vi "FTW-Test-JSON-FloatingPoint.vi"() -> (0 "Test Result":errorcluster)   [LabVIEW 2015]
uses:
  src/json/FTW-JSON-Type.ctl
  src/error/FTW-ERR-ThrowInfo.vi
  src/error/FTW-ERR-ThrowError.vi
  src/error/FTW-ERR-CallChain.vi
  src/string/FTW-STR-ReplaceWhitespace.vi
  src/string/FTW-STR-Array-Delimit.vi
panel:
  out "JSON String (UTF-8)":string
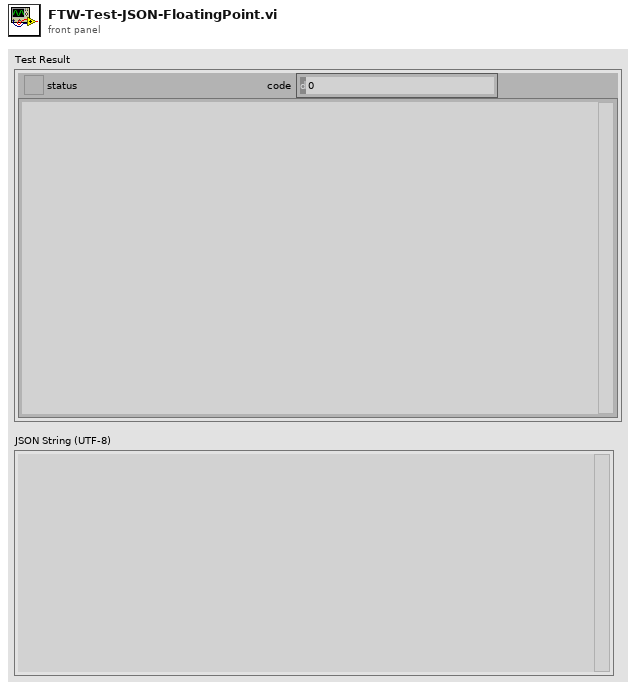
[diagram p1: front panel]
types:
  T1 = typedef "FTW-JSON-Type.ctl" = enum8{"Not Found", "Object", "Array", "String", "Number", "Boolean", "null"}
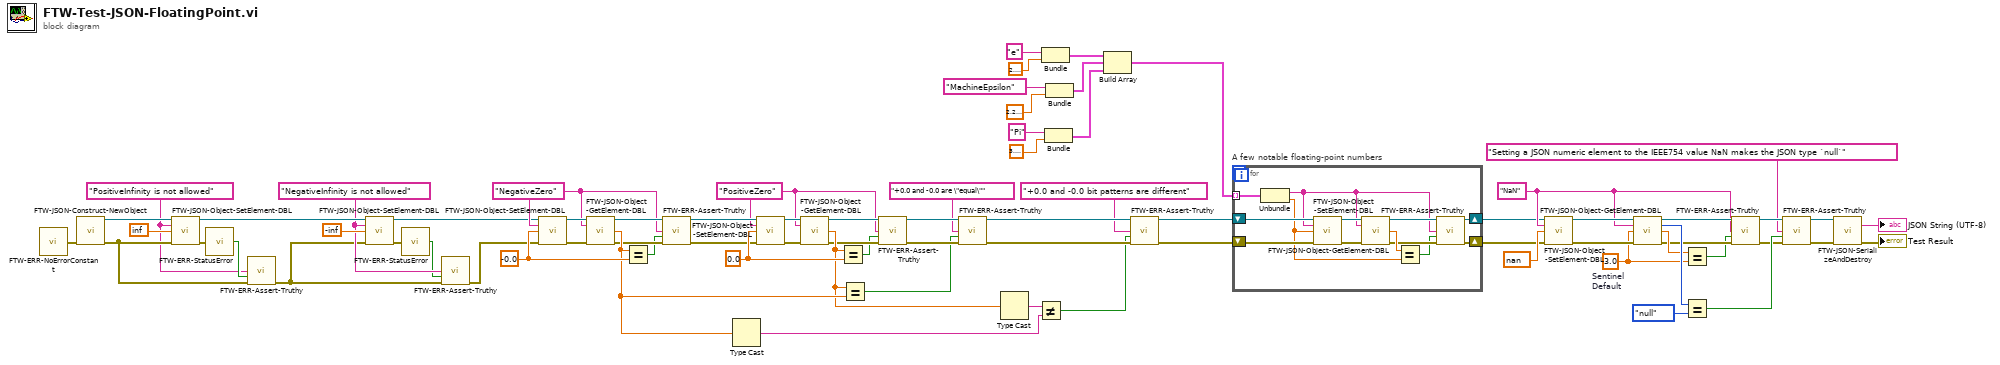
[diagram p0: block diagram]
diagram:
  w54 = 0.0
  w31 = "PositiveZero" ("Key")
  w33 = "NegativeZero" ("Key")
  w53 = -0.0
  w55 = 3.0  # Sentinel Default
  w11 = "NaN" ("Key")
  w41 = "NegativeInfinity is not allowed" ("Key")
  w37 = "PositiveInfinity is not allowed" ("Key")
  n1 = call "FTW-ERR-NoErrorConstant.vi"() -> ("no error"=w70:errorcluster)
  n2 = call "FTW-JSON-Construct-NewObject.vi"("error in"=w70) -> ("JSON Object"=w69:refnum<data-value>, "error out"=w38:errorcluster)  [unwired: 13 in]
  n3 = call "FTW-JSON-Object-SetElement-DBL.vi"("JSON Object"=w69, "Key"=w37, "Value"=inf, "error in"=w38) -> ("JSON Object out"=w67:refnum<data-value>, "error out"=w60:errorcluster)  [unwired: 10 in]
  n4 = call "FTW-ERR-StatusError.vi"("error to check"=w60) -> ("Error?"=w39:bool)
  n5 = call "FTW-ERR-Assert-Truthy.vi"("Assertion"=w37, "Assertion holds true?"=w39, "error in"=w38) -> ("error out"=w36:errorcluster)  [unwired: 12 in]
  n6 = call "FTW-JSON-Object-SetElement-DBL.vi"("JSON Object"=w67, "Key"=w41, "Value"=-inf, "error in"=w36) -> ("JSON Object out"=w14:refnum<data-value>, "error out"=w59:errorcluster)  [unwired: 10 in]
  n7 = call "FTW-ERR-StatusError.vi"("error to check"=w59) -> ("Error?"=w40:bool)
  n8 = call "FTW-ERR-Assert-Truthy.vi"("Assertion"=w41, "Assertion holds true?"=w40, "error in"=w36) -> ("error out"=w13:errorcluster)  [unwired: 12 in]
  n9 = call "FTW-JSON-Object-SetElement-DBL.vi"("JSON Object"=w14, "Key"=w33, "Value"=w53, "error in"=w13) -> ("JSON Object out"=w48:refnum<data-value>, "error out"=w49:errorcluster)  [unwired: 10 in]
  n10 = call "FTW-JSON-Object-GetElement-DBL.vi"("JSON Object"=w48, "Key"=w33, "error in"=w49) -> ("JSON Object out"=w51:refnum<data-value>, "Value"=w46:dbl, "error out"=w35:errorcluster)  [unwired: 9 in, 1 out]
  n11 = Equal?(x=w46, y=w53) -> (x = y?=w32:bool)
  n12 = call "FTW-ERR-Assert-Truthy.vi"("Assertion"=w33, "Assertion holds true?"=w32, "error in"=w35) -> ("error out"=w34:errorcluster)  [unwired: 12 in]
  n13 = Type Cast(x=w46) -> (*(type *) &x=w43:string)  [unwired: 1 in]
  n14 = call "FTW-JSON-Object-SetElement-DBL.vi"("JSON Object"=w51, "Key"=w31, "Value"=w54, "error in"=w34) -> ("JSON Object out"=w50:refnum<data-value>, "error out"=w52:errorcluster)  [unwired: 10 in]
  n15 = call "FTW-JSON-Object-GetElement-DBL.vi"("JSON Object"=w50, "Key"=w31, "error in"=w52) -> ("JSON Object out"=w47:refnum<data-value>, "Value"=w45:dbl, "error out"=w30:errorcluster)  [unwired: 9 in, 1 out]
  n16 = Equal?(x=w45, y=w54) -> (x = y?=w29:bool)
  n17 = Equal?(x=w45, y=w46) -> (x = y?=w27:bool)
  n18 = call "FTW-ERR-Assert-Truthy.vi"("Assertion"=w31, "Assertion holds true?"=w29, "error in"=w30) -> ("error out"=w28:errorcluster)  [unwired: 12 in]
  n19 = call "FTW-ERR-Assert-Truthy.vi"("Assertion"="+0.0 and -0.0 are \"equal\"", "Assertion holds true?"=w27, "error in"=w28) -> ("error out"=w24:errorcluster)  [unwired: 12 in]
  n20 = Type Cast(x=w45) -> (*(type *) &x=w44:string)  [unwired: 1 in]
  n21 = Not Equal?(x=w44, y=w43) -> (x != y?=w22:bool)
  n22 = Bundle("Key"="e", 2.718281828459045) -> (w19:cluster{"Key":string, dbl})  [unwired: 1 in]
  n23 = Bundle("Key"="Pi", 3.141592653589793) -> (w3:cluster{"Key":string, dbl})  [unwired: 1 in]
  n24 = Bundle("Key"="MachineEpsilon", 2.220446049250313e-16) -> (w15:cluster{"Key":string, dbl})  [unwired: 1 in]
  n25 = Build Array(w19, w15, w3) -> (w18:cluster{"Key":string, dbl}[])
  n26 = call "FTW-ERR-Assert-Truthy.vi"("Assertion"="+0.0 and -0.0 bit patterns are different", "Assertion holds true?"=w22, "error in"=w24) -> ("error out"=w23:errorcluster)  [unwired: 12 in]
  n27 = for "A few notable floating-point numbers" {
    shift-right: [w80] -> w2
    shift-left: w47 -> [w78]
    shift-right: [w75] -> w1
    shift-left: w23 -> [w77]
    tunnel: w18 -> [w73] mode=indexing
    n28 = Unbundle(w73) -> ("Key"=w71:string, w72:dbl)
    n29 = call "FTW-JSON-Object-SetElement-DBL.vi"("JSON Object"=w78, "Key"=w71, "Value"=w72, "error in"=w77) -> ("JSON Object out"=w82:refnum<data-value>, "error out"=w81:errorcluster)  [unwired: 10 in]
    n30 = call "FTW-JSON-Object-GetElement-DBL.vi"("JSON Object"=w82, "Key"=w71, "error in"=w81) -> ("JSON Object out"=w80:refnum<data-value>, "Value"=w79:dbl, "error out"=w76:errorcluster)  [unwired: 9 in, 1 out]
    n31 = Equal?(x=w79, y=w72) -> (x = y?=w74:bool)
    n32 = call "FTW-ERR-Assert-Truthy.vi"("Assertion"=w71, "Assertion holds true?"=w74, "error in"=w76) -> ("error out"=w75:errorcluster)  [unwired: 12 in]
  }
  n33 = call "FTW-JSON-Object-SetElement-DBL.vi"("JSON Object"=w2, "Key"=w11, "Value"=nan, "error in"=w1) -> ("JSON Object out"=w63:refnum<data-value>, "error out"=w62:errorcluster)  [unwired: 10 in]
  n34 = call "FTW-JSON-Object-GetElement-DBL.vi"("JSON Object"=w63, "Key"=w11, "Default Value"=w55, "error in"=w62) -> ("JSON Object out"=w61:refnum<data-value>, "JSON Element Type"=w58:T1, "Value"=w56:dbl, "error out"=w12:errorcluster)  [unwired: 8 in]
  n35 = Equal?(x=w56, y=w55) -> (x = y?=w10:bool)
  n36 = Equal?(x=w58, y=FTW-JSON-Type."null") -> (x = y?=w9:bool)
  n37 = call "FTW-ERR-Assert-Truthy.vi"("Assertion"=w11, "Assertion holds true?"=w10, "error in"=w12) -> ("error out"=w7:errorcluster)  [unwired: 12 in]
  n38 = call "FTW-ERR-Assert-Truthy.vi"("Assertion"="Setting a JSON numeric element to the IEEE754 value NaN makes the JSON type `null`", "Assertion holds true?"=w9, "error in"=w7) -> ("error out"=w6:errorcluster)  [unwired: 12 in]
  n39 = call "FTW-JSON-SerializeAndDestroy.vi"("JSON Object"=w61, "error in"=w6) -> ("JSON String (UTF-8)"=→"JSON String (UTF-8)":string, "error out"=→"Test Result":errorcluster)  [unwired: 12 in]
